vi "ScanInterfaceGlobalData.vi"() -> ()   [LabVIEW 2017]
uses:
  Types/StreamInfo.ctl
  Types/ImageInfo.ctl
panel:
  out "CompletedImageBank":T1[](array[typedef])
  out "LastImage":T1
  out "LastStream":T2
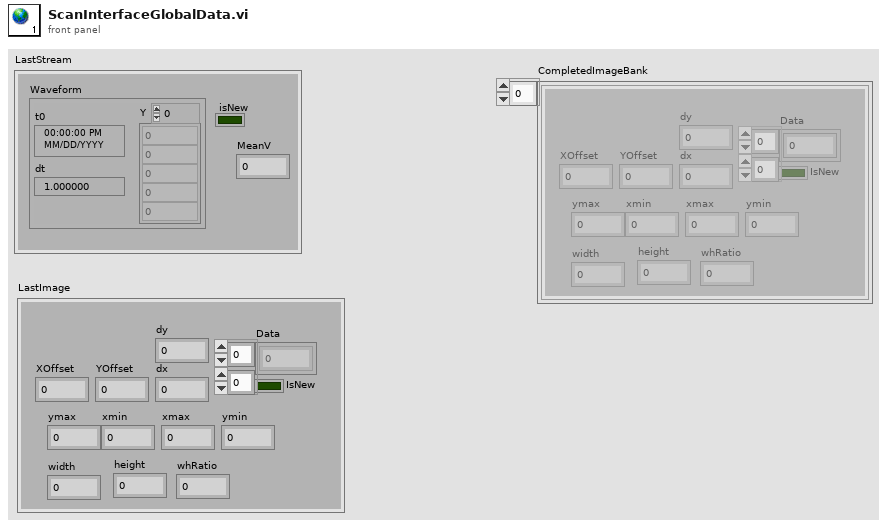
[diagram p1: front panel]
types:
  T1 = typedef "ImageInfo.ctl" = cluster{"IsNew":bool, "Data":dbl[][], "XOffset":dbl, "YOffset":dbl, "dy":dbl, "dx":dbl, "xmin":dbl, "xmax":dbl, "ymin":dbl, "ymax":dbl, "width":dbl, "height":dbl, "whRatio":dbl}
  T2 = typedef "StreamInfo.ctl" = cluster{"Waveform":waveform(dbl), "isNew":bool, "MeanV":dbl}
diagram:
